vi "working_interface.vi"() -> ()   [LabVIEW 2011]
panel:
  in  "delay array 2":dbl[](array[numeric])
  out "Digital Waveform Graph":digitalwaveform(graph)
  in  "command":string="*TRG"
  in  "write command?":bool
  in  "write data":bool
  in  "read delay data":bool
  in  "VISA resource name":refnum<visa-resource-name>
  in  "stop":bool
  # "t0"
  # "t"
  # "A"
  # "B"
  # "C"
  # "D"
  # "E"
  # "F"
  # "G"
  # "H"
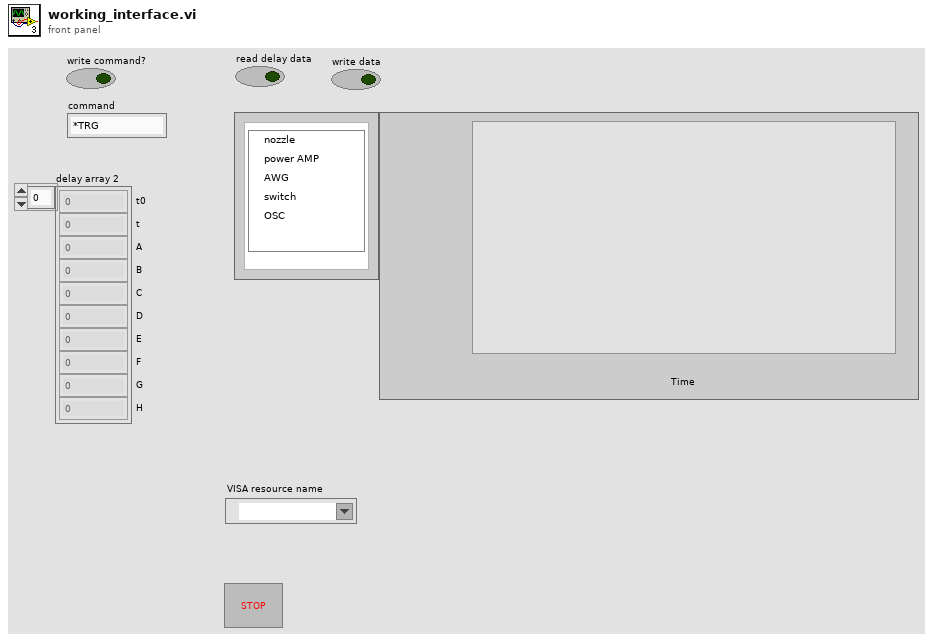
[diagram p1: front panel]
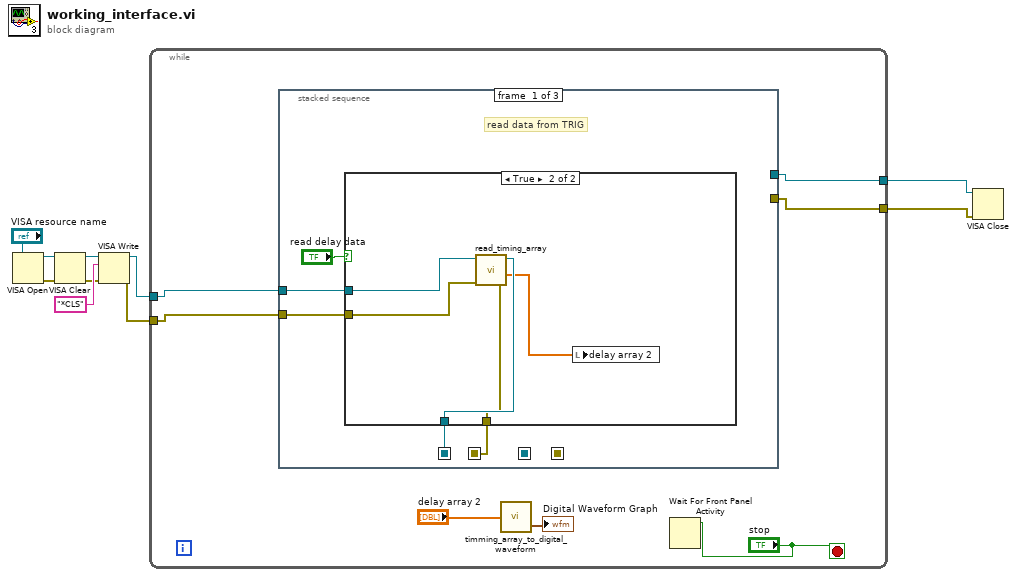
[diagram p0: block diagram]
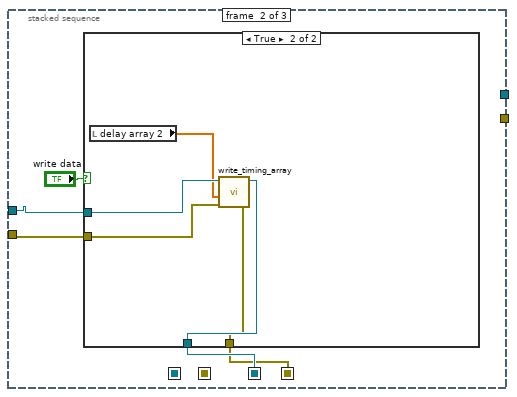
[diagram p3: hidden frame]
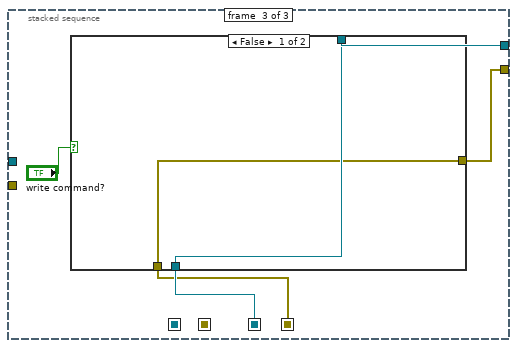
[diagram p5: hidden frame]
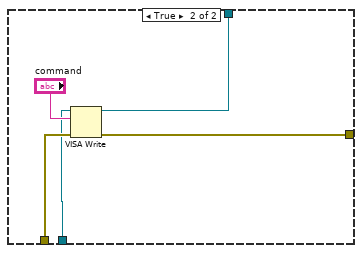
[diagram p6: hidden frame]
diagram:
  n1 = VISA Open(VISA resource name="VISA resource name") -> (VISA resource name=w7:refnum<visa-resource-name>, error out=w8:errorcluster)  [unwired: 4 in]
  n2 = VISA Clear(VISA resource name=w7, error in (no error)=w8) -> (VISA resource name out=w4:refnum<visa-resource-name>, error out=w3:errorcluster)
  n3 = VISA Write(VISA resource name=w4, write buffer="*CLS" ("Query 2"), error in (no error)=w3) -> (VISA resource name out=w6:refnum<visa-resource-name>, error out=w5:errorcluster)  [unwired: 1 out]
  n4 = while {
    tunnel: w6 -> [w14]
    tunnel: w5 -> [w13]
    tunnel: [w16] -> w2
    tunnel: [w15] -> w1
    stop <- "stop" stop-if-true
    n5 = stacked-sequence {
      seq-local: [w20 _ _] -> [_ _ _]
      seq-local: [w19 _ _] -> [_ _ _]
      seq-local: [_ w31 _] -> [_ _ w43]
      seq-local: [_ w30 _] -> [_ _ w42]
      tunnel: w14 -> [w22 w33 _]
      tunnel: w13 -> [w21 w32 _]
      tunnel: [_ _ w45] -> w15
      tunnel: [_ _ w46] -> w16
      frame #0 {
        # "read data from TRIG"
        n6 = case shown="True" "read delay data" {
          tunnel: w22 -> [w23 w29]
          tunnel: w21 -> [w24 w28]
          tunnel: [w23 w27] -> w20
          tunnel: [w24 w26] -> w19
          frame False {
          }
          frame True {
            n7 = call "read_timing_array.vi"("error in"=w28, "VISA resource in"=w29) -> ("error out 2"=w26:errorcluster, "delay array"=w25:dbl[], "VISA resource out"=w27:refnum<visa-resource-name>)  [unwired: 3 in]
            n8 = local write "delay array 2"(w25) -> ()
          }
        }
      }
      frame #1 {
        n9 = case shown="True" "write data" {
          tunnel: w33 -> [w35 w41]
          tunnel: w32 -> [w36 w40]
          tunnel: [w35 w39] -> w31
          tunnel: [w36 w38] -> w30
          frame False {
          }
          frame True {
            n10 = local read "delay array 2"() -> (w37:dbl[])
            n11 = call "write_timing_array.vi"("error in"=w40, "delay array"=w37, "VISA resource in"=w41) -> ("error out 2"=w38:errorcluster, "VISA resource out"=w39:refnum<visa-resource-name>)  [unwired: 3 in]
          }
        }
      }
      frame #2 {
        n12 = case shown="False" "write command?" {
          tunnel: w42 -> [w47 w52]
          tunnel: w43 -> [w48 w51]
          tunnel: [w48 w50] -> w46
          tunnel: [w47 w49] -> w45
          frame False {
          }
          frame True {
            n13 = VISA Write(VISA resource name=w51, write buffer="command", error in (no error)=w52) -> (VISA resource name out=w50:refnum<visa-resource-name>, error out=w49:errorcluster)  [unwired: 1 out]
          }
        }
      }
    }
    n14 = call "timming_array_to_digital_waveform.vi"("timing array"="delay array 2") -> ("digital waveform"=→"Digital Waveform Graph":digitalwaveform)  [unwired: 3 in]
    n15 = Wait For Front Panel Activity(3:"stop") -> ()  [unwired: 2 in, 1 out]
  }
  n16 = VISA Close(VISA resource name=w2, error in (no error)=w1) -> ()  [unwired: 1 out]
